vi "Overlay line segment.vi"(7 "Overlay Coordinates":cluster{"X":sgl, "Y":sgl}[](array[cluster]), 8 "error in (no error)":errorcluster, 9 "Calculated inputs (line)":T1, 10 "User inputs (line)":T2, 11 "Image in":T3) -> (0 "error out":errorcluster, 1 "Overlay coordinates":cluster{"X":sgl, "Y":sgl}[](array[cluster]), 2 "Text origin":cluster{"X":sgl, "Y":sgl}, 3 "Image out":T3, 4 "Out of bounds coord":cluster{"X":sgl, "Y":sgl}[](array[cluster]))   [LabVIEW 2019]
uses:
  <vilib>/vision/Image Controls.llb/IMAQ Image.ctl
  Controls/User inputs (line).ctl
  Controls/Calculated inputs (line).ctl
  <vilib>/vision/NI_Vision_Development_Module.lvlib
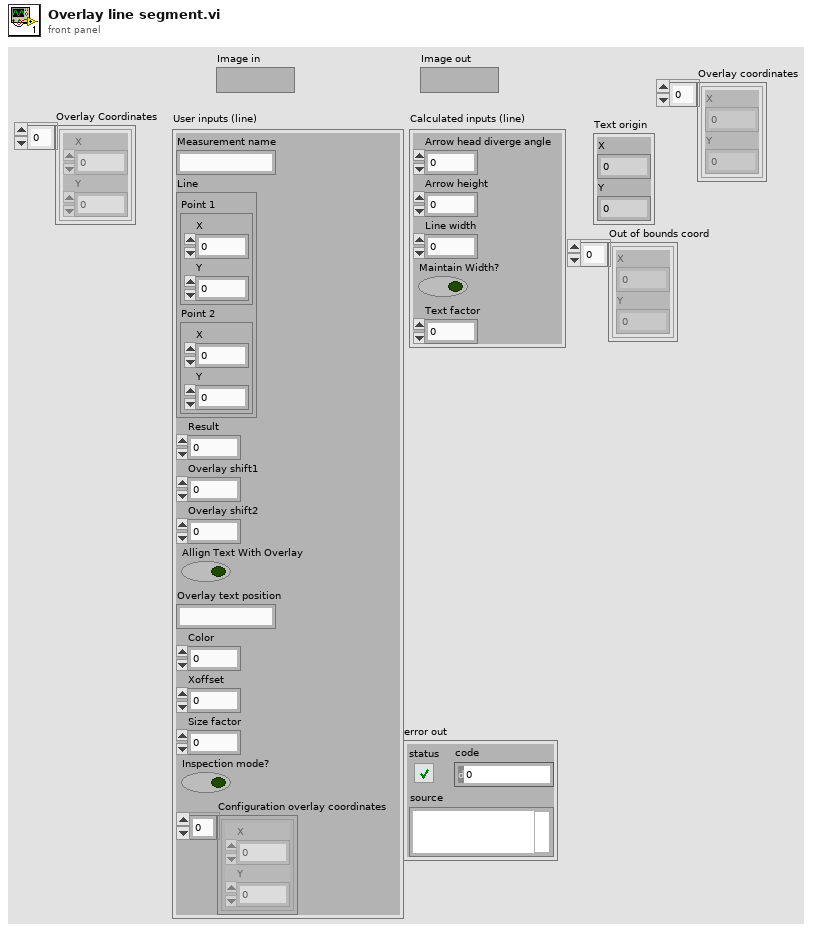
[diagram p1: front panel]
types:
  T1 = typedef "Calculated inputs (line).ctl" = cluster{"Arrow head diverge angle":dbl, "Arrow height":dbl, "Line width":i32, "Maintain Width?":bool, "Text factor":u8}
  T2 = typedef "User inputs (line).ctl" = cluster{"Measurement name":string, "Line":cluster{"Point 1":cluster{"X":sgl, "Y":sgl}, "Point 2":cluster{"X":sgl, "Y":sgl}}, "Result":sgl, "Overlay shift1":dbl, "Overlay shift2":dbl, "Allign Text With Overlay":bool, "Overlay text position":string, "Color":u32, "Xoffset":i32, "Size factor":dbl, "Inspection mode?":bool, "Configuration overlay coordinates":cluster{"X":sgl, "Y":sgl}[]}
  T3 = typedef "IMAQ Image.ctl" = refnum<image>
  T4 = cluster{"Point 1":cluster{"X":sgl, "Y":sgl}, "Point 2":cluster{"X":sgl, "Y":sgl}}
  T5 = cluster{"Desired Font (Application)":enum16{"User-specified Font", "Application Font", "System Font", "Dialog Font"}, "[User-specified Font]":cluster{"Font Name":string, "Size":i16, "Strikeout?":bool, "Italic?":bool, "Underline?":bool, "Outline?":bool, "Shadow?":bool, "Bold?":bool, "Rotation Angle":dbl}, "Horizontal Alignment":i16, "Vertical Alignment":i16}
  T6 = cluster{"Point 1":cluster{"x":dbl, "y":dbl}, "Point 2":cluster{"x":dbl, "y":dbl}}
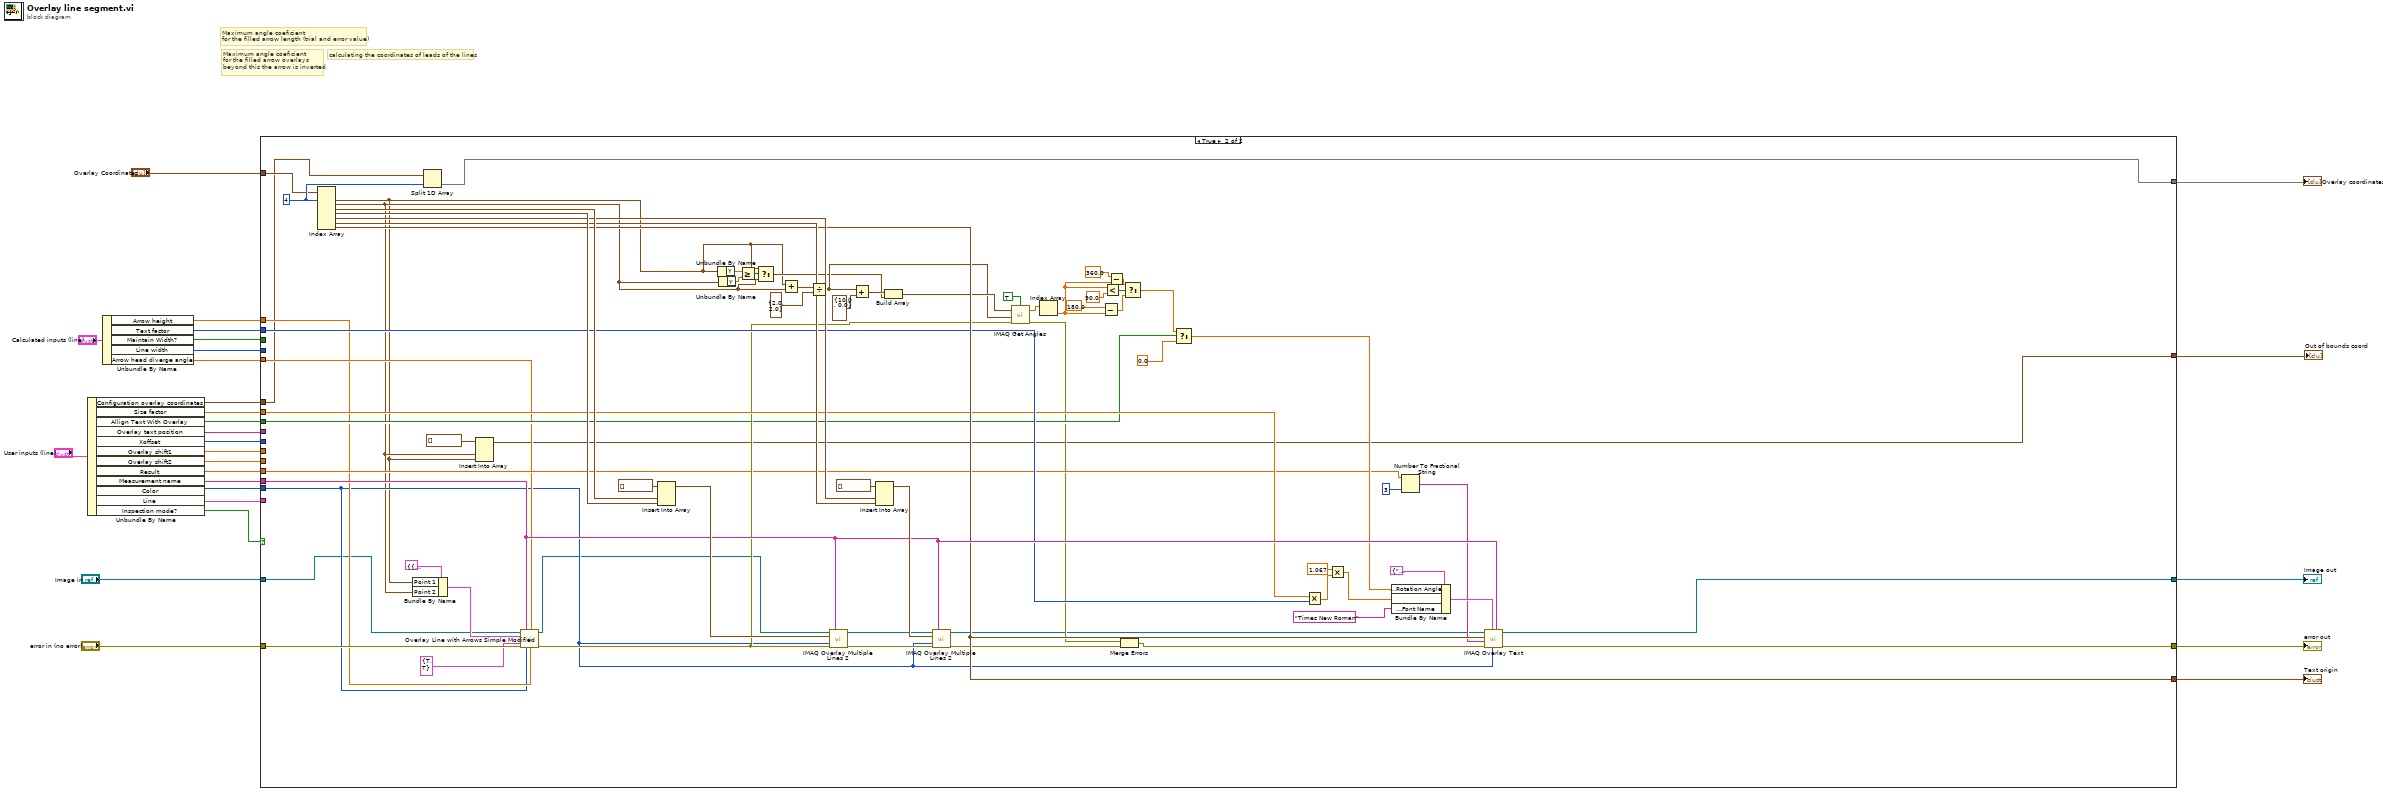
[diagram p0: block diagram]
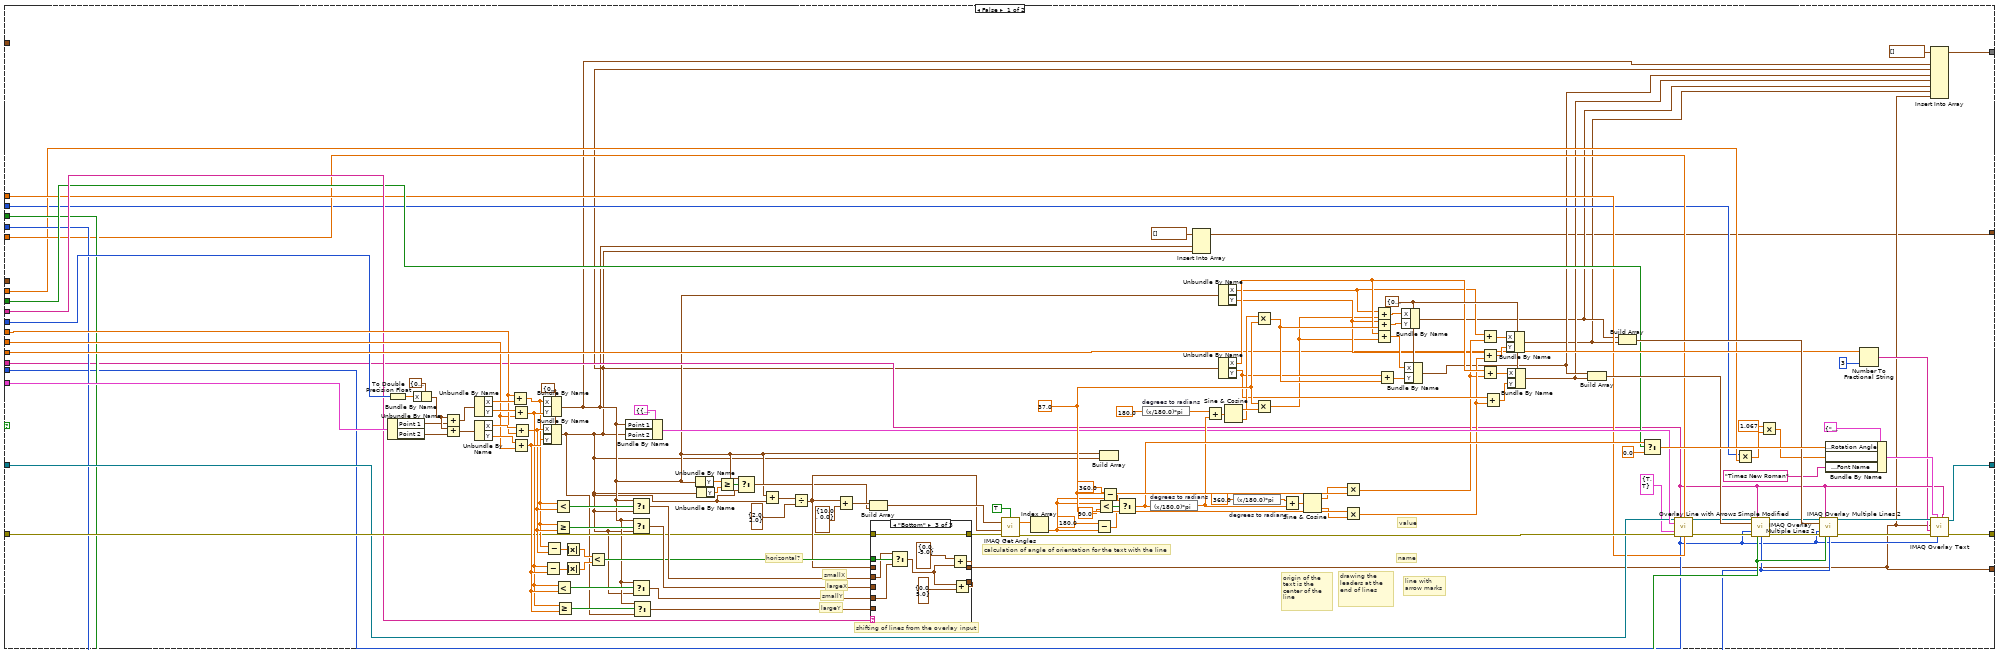
[diagram p2: hidden frame]
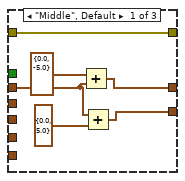
[diagram p3: hidden frame]
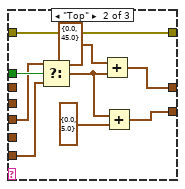
[diagram p4: hidden frame]
diagram:
  # "Maximum angle coeficient\nfor the filled arrow length (trial and error value)"
  # "Maximum angle coeficient\nfor the filled arrow overlays\nbeyond this the arrow is inverted"
  # "calculating the coordinates of leads of the lines"
  n1 = Unbundle By Name("User inputs (line)") -> ("Configuration overlay coordinates"=w3:cluster{"X":sgl, "Y":sgl}[], "Size factor"=w10:dbl, "Allign Text With Overlay"=w15:bool, "Overlay text position"=w16:string, "Xoffset"=w17:i32, "Overlay shift1"=w20:dbl, "Overlay shift2"=w19:dbl, "Result"=w21:sgl, "Measurement name"=w22:string, "Color"=w23:u32, "Line"=w24:T4, "Inspection mode?"=w2:bool)
  n2 = Unbundle By Name("Calculated inputs (line)") -> ("Arrow height"=w14:dbl, "Text factor"=w9:u8, "Maintain Width?"=w13:bool, "Line width"=w12:i32, "Arrow head diverge angle"=w11:dbl)
  n3 = case shown="True" w2 {
    tunnel: [w40 w238] -> w4
    tunnel: [w35 w204] -> w5
    tunnel: "error in (no error)" -> [w134 w252]
    tunnel: "Image in" -> [w67 w194]
    tunnel: w24 -> [w64 _]
    tunnel: w23 -> [w34 w195]
    tunnel: w22 -> [w38 w239]
    tunnel: w21 -> [w63 w202]
    tunnel: w20 -> [w62 _]
    tunnel: w19 -> [w61 _]
    tunnel: w17 -> [w60 _]
    tunnel: w16 -> [w59 _]
    tunnel: w15 -> [w58 w206]
    tunnel: w14 -> [w57 w196]
    tunnel: w13 -> [w56 _]
    tunnel: w12 -> [w55 _]
    tunnel: w11 -> [w54 w197]
    tunnel: w10 -> [w52 w231]
    tunnel: w9 -> [w48 w232]
    tunnel: "Overlay Coordinates" -> [_ w189]
    tunnel: [w33 w237] -> w6
    tunnel: [w43 w188] -> w7
    tunnel: w3 -> [_ w187]
    tunnel: [w28 w183] -> w1
    frame False {
      w124 = cluster{"X":sgl, "Y":sgl} {"X"=0.0, "Y"=0.0} ("x+y")
      w104 = cluster{"X":sgl, "Y":sgl} {"X"=0.0, "Y"=0.0} ("Point 2")
      w158 = sgl 37.0 ("y")
      # "shifting of lines from the overlay input"
      # "largeY"
      # "smallY"
      # "largeX"
      # "smallX"
      # "horizontal?"
      # "drawing the leaders at the end of lines"
      # "origin of the text is the center of the line"
      # "calculation of angle of orientation for the text with the line"
      # "name"
      # "value"
      # "line with\narrow marks"
      n4 = Unbundle By Name(w64) -> ("Point 1"=w120:cluster{"X":sgl, "Y":sgl}, "Point 2"=w122:cluster{"X":sgl, "Y":sgl})
      n5 = To Double Precision Float(number=w60) -> (double precision float=w119:dbl)
      n6 = Bundle By Name(cluster=cluster{"X":sgl, "Y":sgl} {"X"=0.0, "Y"=0.0} ("Angle.Point 2a"), "X"=w119) -> (w121:cluster{"X":sgl, "Y":sgl})
      n7 = Add(x=w121, y=w120) -> (x+y=w130:cluster{"X":sgl, "Y":sgl})
      n8 = Add(x=w121, y=w122) -> (x+y=w129:cluster{"X":sgl, "Y":sgl})
      n9 = Unbundle By Name(w130) -> ("X"=w125:sgl, "Y"=w127:sgl)
      n10 = Unbundle By Name(w129) -> ("X"=w126:sgl, "Y"=w128:sgl)
      n11 = Add(x=w62, y=w125) -> (x+y=w143:dbl)
      n12 = Add(x=w127, y=w61) -> (x+y=w149:dbl)
      n13 = Add(x=w128, y=w61) -> (x+y=w150:dbl)
      n14 = Add(x=w126, y=w62) -> (x+y=w144:dbl)
      n15 = Bundle By Name(cluster=w124, "X"=w143, "Y"=w149) -> (w31:cluster{"X":sgl, "Y":sgl})
      n16 = Bundle By Name(cluster=w124, "X"=w144, "Y"=w150) -> (w30:cluster{"X":sgl, "Y":sgl})
      n17 = Subtract(x=w149, y=w150) -> (x-y=w147:dbl)
      n18 = Subtract(x=w143, y=w144) -> (x-y=w137:dbl)
      n19 = Less?(x=w143, y=w144) -> (x < y?=w142:bool)
      n20 = Greater Or Equal?(x=w143, y=w144) -> (x >= y?=w145:bool)
      n21 = Less?(x=w149, y=w150) -> (x < y?=w148:bool)
      n22 = Greater Or Equal?(x=w149, y=w150) -> (x >= y?=w152:bool)
      n23 = Absolute Value(x=w137) -> (abs(x)=w139:dbl)
      n24 = Absolute Value(x=w147) -> (abs(x)=w138:dbl)
      n25 = Less?(x=w139, y=w138) -> (x < y?=w140:bool)
      n26 = Bundle By Name(cluster=T6 {"Point 1"={"x"=1524.0057373046875, "y"=1020.0}, "Point 2"={"x"=1711.076904296875, "y"=1599.724853515625}} ("Line Coordinates"), "Point 1"=w31, "Point 2"=w30) -> (w117:T6)
      n27 = Select(t=w31, s=w142, f=w30) -> (s? t:f=w141:cluster{"X":sgl, "Y":sgl})
      n28 = Select(t=w31, s=w145, f=w30) -> (s? t:f=w146:cluster{"X":sgl, "Y":sgl})
      n29 = Select(t=w31, s=w148, f=w30) -> (s? t:f=w151:cluster{"X":sgl, "Y":sgl})
      n30 = Select(t=w31, s=w152, f=w30) -> (s? t:f=w153:cluster{"X":sgl, "Y":sgl})
      n31 = Unbundle By Name(w31) -> ("Y"=w70:sgl)
      n32 = Unbundle By Name(w30) -> ("Y"=w71:sgl)
      n33 = Greater Or Equal?(x=w70, y=w71) -> (x >= y?=w72:bool)
      n34 = Select(t=w31, s=w72, f=w30) -> (s? t:f=w42:cluster{"X":sgl, "Y":sgl})
      n35 = Add(x=w31, y=w30) -> (x+y=w68:cluster{"X":sgl, "Y":sgl})
      n36 = Divide(x=w68, y=cluster{"X":sgl, "Y":sgl} {"X"=2.0, "Y"=2.0}) -> (x/y=w136:cluster{"X":sgl, "Y":sgl})
      n37 = Add(x=w136, y=cluster{"X":sgl, "Y":sgl} {"X"=10.0, "Y"=0.0}) -> (x+y=w80:cluster{"X":sgl, "Y":sgl})
      n38 = Build Array(w80, w42) -> (w154:cluster{"X":sgl, "Y":sgl}[])
      n39 = case shown="\"Bottom\"" w59 {
        tunnel: w134 -> [w164 w173 w182]
        tunnel: [w164 w173 w182] -> w135
        tunnel: [w160 w165 w179] -> w33
        tunnel: w136 -> [w161 _ _]
        tunnel: [w159 w170 w178] -> _
        tunnel: w140 -> [_ w169 w177]
        tunnel: w141 -> [_ _ w176]
        tunnel: w146 -> [_ w168 _]
        tunnel: w151 -> [_ _ w175]
        tunnel: w153 -> [_ w167 _]
        frame "Middle", Default {
          n40 = Add(x=cluster{"X":sgl, "Y":sgl} {"X"=0.0, "Y"=-5.0} ("y"), y=w161) -> (x+y=w160:cluster{"X":sgl, "Y":sgl})
          n41 = Add(x=w161, y=cluster{"X":sgl, "Y":sgl} {"X"=0.0, "Y"=5.0}) -> (x+y=w159:cluster{"X":sgl, "Y":sgl})
        }
        frame "Top" {
          n42 = Select(t=w168, s=w169, f=w167) -> (s? t:f=w166:cluster{"X":sgl, "Y":sgl})
          n43 = Add(x=cluster{"X":sgl, "Y":sgl} {"X"=0.0, "Y"=45.0} ("y"), y=w166) -> (x+y=w165:cluster{"X":sgl, "Y":sgl})
          n44 = Add(x=w166, y=cluster{"X":sgl, "Y":sgl} {"X"=0.0, "Y"=5.0}) -> (x+y=w170:cluster{"X":sgl, "Y":sgl})
        }
        frame "Bottom" {
          n45 = Select(t=w176, s=w177, f=w175) -> (s? t:f=w174:cluster{"X":sgl, "Y":sgl})
          n46 = Add(x=cluster{"X":sgl, "Y":sgl} {"X"=0.0, "Y"=-5.0} ("y"), y=w174) -> (x+y=w179:cluster{"X":sgl, "Y":sgl})
          n47 = Add(x=w174, y=cluster{"X":sgl, "Y":sgl} {"X"=0.0, "Y"=5.0}) -> (x+y=w178:cluster{"X":sgl, "Y":sgl})
        }
      }
      n48 = call "IMAQ Get Angles"("error in (no error)"=w135, "Vertex"=w136, "Points"=w154, "Use Vertex (No)"=TRUE) -> ("error out"=w84:errorcluster, "Angles (deg)"=w76:sgl[])  [unwired: 1 in, 1 out]
      n49 = Index Array(array=w76) -> (element=w109:sgl)  [unwired: 1 in]
      n50 = Subtract(x=sgl 180.0 ("y"), y=w109) -> (x-y=w82:sgl)
      n51 = Less?(x=w109, y=sgl 90.0) -> (x < y?=w77:bool)
      n52 = Build Array(w31, w30) -> ()  [unwired: 1 out]
      n53 = Subtract(x=sgl 360.0 ("y"), y=w109) -> (x-y=w79:sgl)
      n54 = Select(t=w79, s=w77, f=w82) -> (s? t:f=w132:sgl)
      n55 = expression code="(x/180.0)*pi" "degrees to radians"(sgl 180.0 ("x")) -> (w111:sgl)
      n56 = expression code="(x/180.0)*pi" "degrees to radians"(w132) -> (w123:sgl)
      n57 = Insert Into Array(array=cluster{"X":sgl, "Y":sgl}[] [], new element #1=w31, new element #2=w30) -> (w28:cluster{"X":sgl, "Y":sgl}[])  [unwired: 1 in]
      n58 = Add(x=w111, y=w123) -> (x+y=w85:sgl)
      n59 = Unbundle By Name(w31) -> ("X"=w90:sgl, "Y"=w91:sgl)
      n60 = Unbundle By Name(w30) -> ("X"=w94:sgl, "Y"=w95:sgl)
      n61 = Sine & Cosine(0:w85) -> (1:w156:sgl, 2:w155:sgl)
      n62 = expression code="(x/180.0)*pi" "degrees to radians"(sgl 360.0 ("x")) -> (w112:sgl)
      n63 = Multiply(x=w155, y=w158) -> (x*y=w157:sgl)
      n64 = Multiply(x=w158, y=w156) -> (x*y=w86:sgl)
      n65 = Add(x=w112, y=w123) -> (x+y=w87:sgl)
      n66 = Sine & Cosine(0:w87) -> (1:w89:sgl, 2:w88:sgl)
      n67 = Multiply(x=w89, y=w158) -> (x*y=w92:sgl)
      n68 = Multiply(x=w158, y=w88) -> (x*y=w93:sgl)
      n69 = Add(x=w90, y=w86) -> (x+y=w97:sgl)
      n70 = Add(x=w91, y=w157) -> (x+y=w96:sgl)
      n71 = Add(x=w94, y=w86) -> (x+y=w98:sgl)
      n72 = Add(x=w95, y=w157) -> (x+y=w99:sgl)
      n73 = Bundle By Name(cluster=w104, "X"=w97, "Y"=w96) -> (w45:cluster{"X":sgl, "Y":sgl})
      n74 = Bundle By Name(cluster=w104, "X"=w98, "Y"=w99) -> (w47:cluster{"X":sgl, "Y":sgl})
      n75 = Add(x=w90, y=w92) -> (x+y=w100:sgl)
      n76 = Add(x=w91, y=w93) -> (x+y=w101:sgl)
      n77 = Add(x=w94, y=w92) -> (x+y=w102:sgl)
      n78 = Add(x=w95, y=w93) -> (x+y=w103:sgl)
      n79 = Bundle By Name(cluster=w104, "X"=w100, "Y"=w101) -> (w44:cluster{"X":sgl, "Y":sgl})
      n80 = Bundle By Name(cluster=w104, "X"=w102, "Y"=w103) -> (w46:cluster{"X":sgl, "Y":sgl})
      n81 = Build Array(w47, w46) -> (w114:cluster{"X":sgl, "Y":sgl}[])
      n82 = Build Array(w45, w44) -> (w115:cluster{"X":sgl, "Y":sgl}[])
      n83 = Select(t=w132, s=w58, f=sgl 0.0 ("s? t:f")) -> (s? t:f=w133:sgl)
      n84 = call "Overlay Line with Arrows Simple Modified.vi"("Image In"=w67, "Group"=w38, "Angle Coefficient"=w54, "Line Coordinates"=w117, "Arrows"=cluster{"Start point":bool, "End point":bool} {"Start point"=TRUE, "End point"=TRUE}, "error in"=w84, "Color"=w34, "Height Coefficient"=w57) -> ("Image Out"=w106:T3, "error out"=w105:errorcluster)  [unwired: 6 in]
      n85 = Multiply(x=w48, y=w52) -> (x*y=w51:dbl)
      n86 = call "IMAQ Overlay Multiple Lines 2"("Image"=w106, "Group"=w38, "Line End Points"=w114, "Color"=w34, "error in (no error)"=w105, "Maintain Width?"=w56, "Width"=w55) -> ("Image Out"=w108:T3, "error out"=w107:errorcluster)  [unwired: 7 in]
      n87 = Multiply(x=1.067, y=w51) -> (x*y=w49:dbl)
      n88 = call "IMAQ Overlay Multiple Lines 2"("Image"=w108, "Group"=w38, "Line End Points"=w115, "Color"=w34, "error in (no error)"=w107, "Maintain Width?"=w56, "Width"=w55) -> ("Image Out"=w37:T3, "error out"=w41:errorcluster)  [unwired: 7 in]
      n89 = Bundle By Name(cluster=T5 {"Desired Font (Application)"=enum."User-specified Font", "[User-specified Font]"={"Font Name"="", "Size"=40, "Strikeout?"=FALSE, "Italic?"=FALSE, "Underline?"=FALSE, "Outline?"=FALSE, "Shadow?"=FALSE, "Bold?"=TRUE, "Rotation Angle"=0.0}, "Horizontal Alignment"=1, "Vertical Alignment"=2} ("Font, Size & Style"), "[User-specified Font].Rotation Angle"=w133, "[User-specified Font].Size"=w49, "[User-specified Font].Font Name"="Times New Roman") -> (w39:T5)
      n90 = Number To Fractional String(number=w63, precision (6)=i16 3) -> (F-format string=w36:string)  [unwired: 2 in]
      n91 = Insert Into Array(array=cluster{"X":sgl, "Y":sgl}[] [], new element #1=w31, new element #2=w30, new element #3=w47, new element #4=w46, new element #5=w45, new element #6=w44, new element #7=w33) -> (w43:cluster{"X":sgl, "Y":sgl}[])  [unwired: 1 in]
      n92 = call "IMAQ Overlay Text"("Group"=w38, "Text Color (black)"=w34, "Font, Size & Style"=w39, "error in (no error)"=w41, "String"=w36, "Origin"=w33, "Image"=w37) -> ("error out"=w40:errorcluster, "Image Out"=w35:T3)  [unwired: 3 in]
    }
    frame True {
      w190 = 4 ("index")
      n93 = Index Array(array=w189, index #1=w190) -> (element #1=w185:cluster{"X":sgl, "Y":sgl}, element #2=w186:cluster{"X":sgl, "Y":sgl}, element #3=w247:cluster{"X":sgl, "Y":sgl}, element #4=w245:cluster{"X":sgl, "Y":sgl}, element #5=w242:cluster{"X":sgl, "Y":sgl}, element #6=w241:cluster{"X":sgl, "Y":sgl}, element #7=w237:cluster{"X":sgl, "Y":sgl})  [unwired: 6 in]
      n94 = Bundle By Name(cluster=T6 {"Point 1"={"x"=0.0, "y"=0.0}, "Point 2"={"x"=0.0, "y"=0.0}} ("Line Coordinates"), "Point 1"=w185, "Point 2"=w186) -> (w249:T6)
      n95 = Split 1D Array(array=w187, index=w190) -> (second subarray=w188:cluster{"X":sgl, "Y":sgl}[])  [unwired: 1 out]
      n96 = Insert Into Array(array=cluster{"X":sgl, "Y":sgl}[] [], new element #1=w186, new element #2=w185) -> (w183:cluster{"X":sgl, "Y":sgl}[])  [unwired: 1 in]
      n97 = call "Overlay Line with Arrows Simple Modified.vi"("Image In"=w194, "Group"=w239, "Angle Coefficient"=w197, "Line Coordinates"=w249, "Arrows"=cluster{"Start point":bool, "End point":bool} {"Start point"=TRUE, "End point"=TRUE}, "error in"=w252, "Color"=w195, "Height Coefficient"=w196) -> ("Image Out"=w193:T3, "error out"=w211:errorcluster)  [unwired: 6 in]
      n98 = Insert Into Array(array=cluster{"X":sgl, "Y":sgl}[] [], new element #1=w247, new element #2=w245) -> (w244:cluster{"X":sgl, "Y":sgl}[])  [unwired: 1 in]
      n99 = Unbundle By Name(w185) -> ("Y"=w214:sgl)
      n100 = Unbundle By Name(w186) -> ("Y"=w215:sgl)
      n101 = Greater Or Equal?(x=w214, y=w215) -> (x >= y?=w216:bool)
      n102 = Select(t=w185, s=w216, f=w186) -> (s? t:f=w223:cluster{"X":sgl, "Y":sgl})
      n103 = Add(x=w185, y=w186) -> (x+y=w212:cluster{"X":sgl, "Y":sgl})
      n104 = Divide(x=w212, y=cluster{"X":sgl, "Y":sgl} {"X"=2.0, "Y"=2.0}) -> (x/y=w229:cluster{"X":sgl, "Y":sgl})
      n105 = call "IMAQ Overlay Multiple Lines 2"("Image"=w193, "Group"=w239, "Line End Points"=w244, "Color"=w195, "error in (no error)"=w211) -> ("Image Out"=w192:T3, "error out"=w251:errorcluster)  [unwired: 9 in]
      n106 = Add(x=w229, y=cluster{"X":sgl, "Y":sgl} {"X"=10.0, "Y"=0.0}) -> (x+y=w224:cluster{"X":sgl, "Y":sgl})
      n107 = Insert Into Array(array=cluster{"X":sgl, "Y":sgl}[] [], new element #1=w242, new element #2=w241) -> (w240:cluster{"X":sgl, "Y":sgl}[])  [unwired: 1 in]
      n108 = Build Array(w224, w223) -> (w230:cluster{"X":sgl, "Y":sgl}[])
      n109 = call "IMAQ Overlay Multiple Lines 2"("Image"=w192, "Group"=w239, "Line End Points"=w240, "Color"=w195, "error in (no error)"=w251) -> ("Image Out"=w191:T3, "error out"=w200:errorcluster)  [unwired: 9 in]
      n110 = call "IMAQ Get Angles"("error in (no error)"=w211, "Vertex"=w229, "Points"=w230, "Use Vertex (No)"=TRUE) -> ("error out"=w198:errorcluster, "Angles (deg)"=w219:sgl[])  [unwired: 1 in, 1 out]
      n111 = Index Array(array=w219) -> (element=w228:sgl)  [unwired: 1 in]
      n112 = Subtract(x=sgl 180.0 ("y"), y=w228) -> (x-y=w226:sgl)
      n113 = Less?(x=w228, y=sgl 90.0) -> (x < y?=w220:bool)
      n114 = Subtract(x=sgl 360.0 ("y"), y=w228) -> (x-y=w222:sgl)
      n115 = Merge Errors(w198, w200) -> (w199:errorcluster)
      n116 = Select(t=w222, s=w220, f=w226) -> (s? t:f=w208:sgl)
      n117 = Select(t=w208, s=w206, f=sgl 0.0) -> (s? t:f=w205:sgl)
      n118 = Multiply(x=w231, y=w232) -> (x*y=w235:dbl)
      n119 = Multiply(x=1.067, y=w235) -> (x*y=w233:dbl)
      n120 = Bundle By Name(cluster=T5 {"Desired Font (Application)"=enum."User-specified Font", "[User-specified Font]"={"Font Name"="", "Size"=40, "Strikeout?"=FALSE, "Italic?"=FALSE, "Underline?"=FALSE, "Outline?"=FALSE, "Shadow?"=FALSE, "Bold?"=TRUE, "Rotation Angle"=0.0}, "Horizontal Alignment"=1, "Vertical Alignment"=2} ("Font, Size & Style"), "[User-specified Font].Rotation Angle"=w205, "[User-specified Font].Size"=w233, "[User-specified Font].Font Name"="Times New Roman") -> (w209:T5)
      n121 = Number To Fractional String(number=w202, precision (6)=i16 3) -> (F-format string=w201:string)  [unwired: 2 in]
      n122 = call "IMAQ Overlay Text"("Group"=w239, "Text Color (black)"=w195, "Font, Size & Style"=w209, "error in (no error)"=w199, "String"=w201, "Origin"=w237, "Image"=w191) -> ("error out"=w238:errorcluster, "Image Out"=w204:T3)  [unwired: 3 in]
    }
  }
  "error out" <- w4
  "Image out" <- w5
  "Text origin" <- w6
  "Overlay coordinates" <- w7
  "Out of bounds coord" <- w1
